vi "ConfigDMM.vi"(8 "error in (no error)":errorcluster, 11 "Input parameters":T1={"Measurement type"=enum."Test", "Sensor type"=enum."HPK_8in_256", "Identifier"="test.txt", "Open after execution?"=FALSE, "Plot after execution?"=FALSE, "Display channel"=0, "Voltage Delay (s)"=0.5, "Switch Delay (s)"=0.01, "VISA resource name source"="", "VISA resource name DMM"="", "VISA resource name LCR"="", "Compliance  Level (uA)"=10.0, "Voltage Limit (V)"=1000.0, "Data storage location"="", "Scan voltages"="", "Use source as DMM?"=FALSE, "Single channel?"=FALSE, "LCR signal frequenzy (Hz)"=10.0, "DMM device"=enum."Keithley2001", "Sampling number"=1, "Use env. sensors on"=enum."Sensirion sht1x/7x"} {"Voltage Limit (V)" format="%#_13g"; "Voltage Delay (s)" format="%#_13g"; "Switch Delay (s)" format="%#_13g"}) -> (0 "error out":errorcluster)   [LabVIEW 2016]
uses:
  Input_parameters.ctl
  instr.lib/ke2001/KE2001.LLB/Keith 2001 Reset / Preset.vi
  instr.lib/Keithley 2450/Keithley 2450.lvlib
panel:
  out "VISA resource name out":refnum<visa-resource-name>
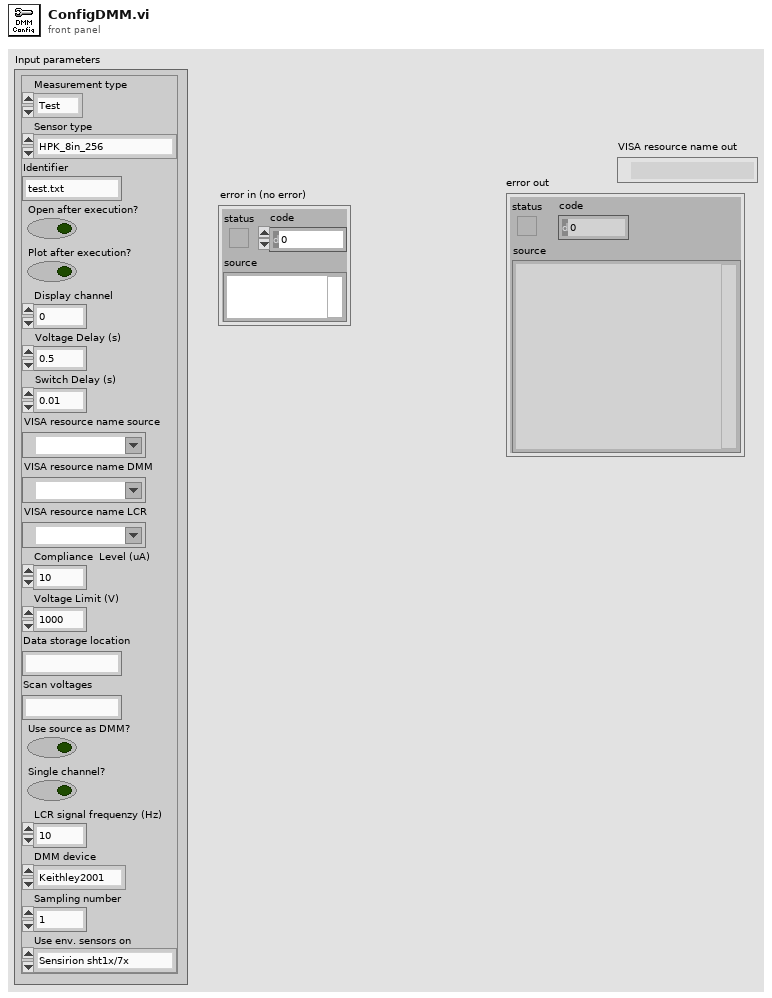
[diagram p1: front panel]
types:
  T1 = typedef "Input_parameters.ctl" = cluster{"Measurement type":enum16{"IV", "CV", "Test"}, "Sensor type":enum16{"HPK_6in_135", "HPK_8in_256", "INF_8in_256", "Diode", "HPK_6in_256", "Test capacitances"}, "Identifier":string, "Open after execution?":bool, "Plot after execution?":bool, "Display channel":i32, "Voltage Delay (s)":dbl, "Switch Delay (s)":dbl, "VISA resource name source":refnum<visa-resource-name>, "VISA resource name DMM":refnum<visa-resource-name>, "VISA resource name LCR":refnum<visa-resource-name>, "Compliance  Level (uA)":dbl, "Voltage Limit (V)":dbl, "Data storage location":string, "Scan voltages":string, "Use source as DMM?":bool, "Single channel?":bool, "LCR signal frequenzy (Hz)":dbl, "DMM device":enum16{"Keithley2001", "Keithley2450", "Keithley2410", "Keithley6487"}, "Sampling number":i32, "Use env. sensors on":enum16{"Sensirion sht1x/7x", "Switch Matrix", "Probecard"}}
  T2 = enum16{"Keithley2001", "Keithley2450", "Keithley2410", "Keithley6487"}
  T3 = enum16{"Auto On", "2e-9", "2e-8", "2e-7", "2e-6", "2e-5", "2e-4", "2e-3", "2e-2"}
  T4 = cluster{"error":bool, "code":i32, "source":string}
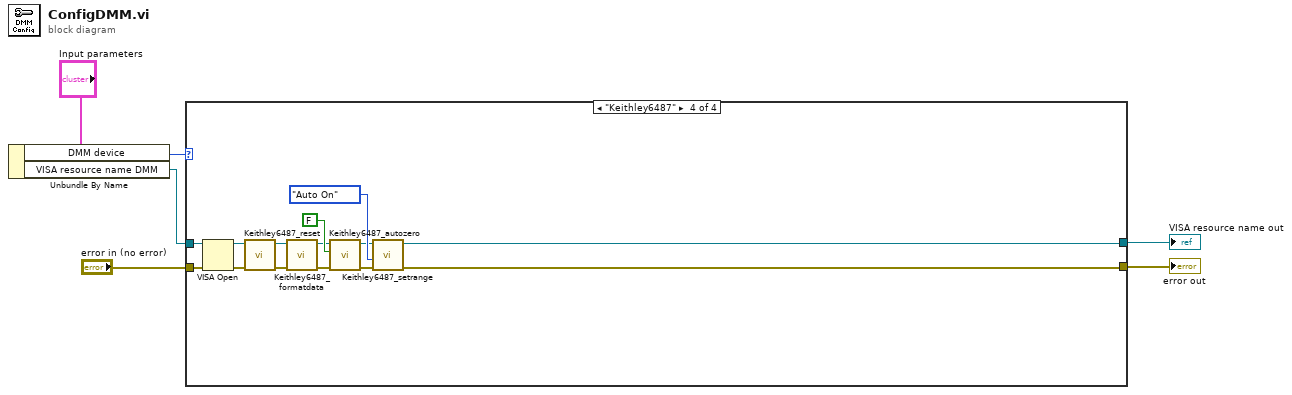
[diagram p0: block diagram]
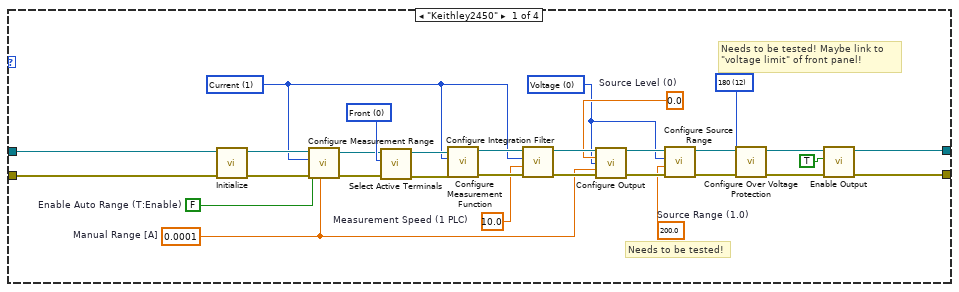
[diagram p2: hidden frame]
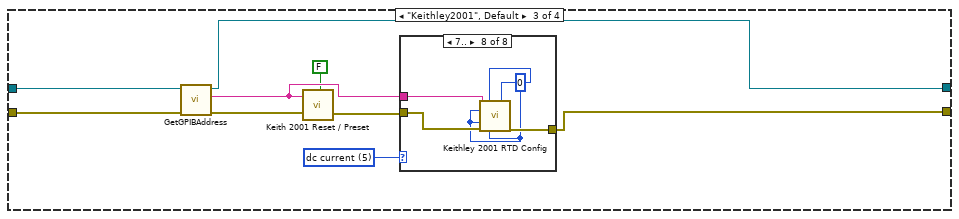
[diagram p4: hidden frame]
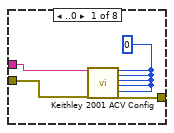
[diagram p5: hidden frame]
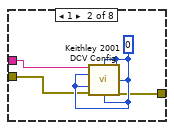
[diagram p6: hidden frame]
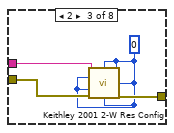
[diagram p7: hidden frame]
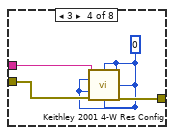
[diagram p8: hidden frame]
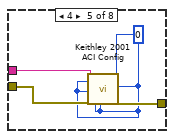
[diagram p9: hidden frame]
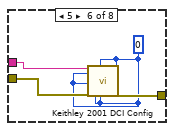
[diagram p10: hidden frame]
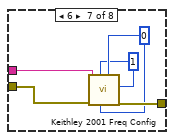
[diagram p11: hidden frame]
diagram:
  n1 = Unbundle By Name("Input parameters") -> ("DMM device"=w3:T2, "VISA resource name DMM"=w2:refnum<visa-resource-name>)
  n2 = case shown="\"Keithley6487\"" w3 {
    tunnel: w2 -> [w36 w38 w45 w83]
    tunnel: "error in (no error)" -> [w35 w37 w44 w84]
    tunnel: [w7 w37 w46 w85] -> w5
    tunnel: [w8 w38 w43 w86] -> w4
    frame "Keithley2450" {
      w12 = u16 12 items=["None", "2", "5", "10", "20", "40", "60", "80", "100", "120", "140", "160", "180"] ("Voltage Limit (0)")
      w15 = 200.0  # Source Range (1.0)
      w20 = 0.0  # Source Level (0)
      w16 = u16 0 items=["Voltage", "Current"] ("Source Mode  (0: Voltage)")
      w23 = 10.0  # Measurement Speed (1 PLC)
      w24 = u16 1 items=["Volts", "Current", "Resistance"] ("Function (0: Volts)")
      w19 = 0.0001  # Manual Range [A]
      w27 = FALSE  # Enable Auto Range (T:Enable)
      w32 = u16 0 items=["Front", "Rear"] ("Active Terminals (0: Front)")
      # "Needs to be tested! Maybe link to \n\"voltage limit\" of front panel!"
      # "Needs to be tested!"
      n3 = call "Initialize.vi"("error in (no error)"=w35, "VISA resource name"=w36) -> ("error out"=w33:errorcluster, "VISA resource name out"=w34:refnum<visa-resource-name>)  [unwired: 8 in]
      n4 = call "Configure Measurement Range.vi"("Manual Range (1.0)"=w19, "error in (no error)"=w33, "Enable Auto Range (T:Enable)"=w27, "Function (0: Volts)"=w24, "VISA resource name"=w34) -> ("error out"=w31:errorcluster, "VISA resource name out"=w28:refnum<visa-resource-name>)  [unwired: 5 in]
      n5 = call "Select Active Terminals.vi"("error in (no error)"=w31, "Active Terminals (0: Front)"=w32, "VISA resource name"=w28) -> ("error out"=w30:errorcluster, "VISA resource name out"=w29:refnum<visa-resource-name>)  [unwired: 7 in]
      n6 = call "Configure Measurement Function.vi"("error in (no error)"=w30, "Function (0: Volts)"=w24, "VISA resource name"=w29) -> ("error out"=w25:errorcluster, "VISA resource name out"=w26:refnum<visa-resource-name>)  [unwired: 7 in]
      n7 = call "Configure Integration Filter.vi"("error in (no error)"=w25, "Measurement Speed (1 PLC)"=w23, "Function (0: Volts)"=w24, "VISA resource name"=w26) -> ("error out"=w21:errorcluster, "VISA resource name out"=w22:refnum<visa-resource-name>)  [unwired: 6 in]
      n8 = call "Configure Output.vi"("VISA resource name"=w22, "Source Level (0)"=w20, "Source Mode  (0: Voltage)"=w16, "Source Limit Level (0.1)"=w19, "error in (no error)"=w21) -> ("VISA resource name out"=w17:refnum<visa-resource-name>, "error out"=w18:errorcluster)  [unwired: 9 in]
      n9 = call "Configure Source Range.vi"("error in (no error)"=w18, "Source Range (1.0)"=w15, "Function (0: Volts)"=w16, "VISA resource name"=w17) -> ("error out"=w14:errorcluster, "VISA resource name out"=w13:refnum<visa-resource-name>)  [unwired: 6 in]
      n10 = call "Configure Over Voltage Protection.vi"("error in (no error)"=w14, "Voltage Limit (0)"=w12, "VISA resource name"=w13) -> ("error out"=w10:errorcluster, "VISA resource name out"=w9:refnum<visa-resource-name>)  [unwired: 7 in]
      n11 = call "Enable Output.vi"("error in (no error)"=w10, "Enable Output (T: Enable)"=TRUE, "VISA resource name"=w9) -> ("error out"=w7:errorcluster, "VISA resource name out"=w8:refnum<visa-resource-name>)  [unwired: 7 in]
    }
    frame "Keithley2410" {
    }
    frame "Keithley2001", Default {
      w47 = u16 5 items=["ac voltage", "dc voltage", "2-wire resistance", "4-wire resistance", "ac current", "dc current", "frequency", "temperature"] ("function (Vdc:1)")
      n12 = call "GetGPIBAddress.vi"("error in (no error)"=w44, "VISA resource name"=w45) -> ("error out"=w42:errorcluster, "GPIB address"=w41:string, "VISA resource name out"=w43:refnum<visa-resource-name>)  [unwired: 7 in]
      n13 = call "Keith 2001 Reset / Preset.vi"("reset/preset"=FALSE, "error in"=w42, "GPIB address"=w41) -> ("error out"=w40:T4)
      n14 = case shown="7.." w47 {
        tunnel: w40 -> [w50 w54 w58 w62 w66 w70 w75 w79]
        tunnel: w41 -> [w48 w53 w57 w61 w65 w68 w74 w78]
        tunnel: [w49 w52 w59 w63 w67 w71 w76 w80] -> w46
        frame ..0 {
          w51 = u16 0
          n15 = call "Keithley 2001 ACV Config.vi"("GPIB address"=w48, "integration time (0:auto)"=w51, "integ. value"=w51, "range (auto:0)"=w51, "error in"=w50, "resolution (4.5 digits:3)"=w51, "reference (off:0)"=w51, "digital filter (off:0)"=w51, "advanced filter (off:0)"=w51, "detector (rms:0)"=w51) -> ("error out"=w49:T4)  [unwired: 9 in]
        }
        frame 1 {
          w55 = u16 0
          n16 = call "Keithley 2001 DCV Config.vi"("GPIB address"=w53, "range (auto:0)"=w55, "digital filter (off:0)"=w55, "integration time (0:auto)"=w55, "advanced filter (off:0)"=w55, "resolution (4.5 digits:3)"=w55, "error in"=w54, "reference value (volts)"=w55) -> ("error out"=w52:T4)  [unwired: 7 in]
        }
        frame 2 {
          w56 = u16 0
          n17 = call "Keithley 2001 2-W Res Config.vi"("GPIB address"=w57, "range (auto:0)"=w56, "digital filter (off:0)"=w56, "integration time (0:auto)"=w56, "advanced filter (off:0)"=w56, "resolution (4.5 digits:3)"=w56, "error in"=w58, "reference value (ohms)"=w56) -> ("error out"=w59:T4)  [unwired: 7 in]
        }
        frame 3 {
          w60 = u16 0
          n18 = call "Keithley 2001 4-W Res Config.vi"("GPIB address"=w61, "range (auto:0)"=w60, "digital filter (off:0)"=w60, "integration time (0:auto)"=w60, "advanced filter (off:0)"=w60, "resolution (4.5 digits:3)"=w60, "error in"=w62, "reference value (ohms)"=w60) -> ("error out"=w63:T4)  [unwired: 7 in]
        }
        frame 4 {
          w64 = u16 0
          n19 = call "Keithley 2001 ACI Config.vi"("GPIB address"=w65, "integration time (0:auto)"=w64, "range (auto:0)"=w64, "error in"=w66, "resolution (4.5 digits:3)"=w64, "digital filter (off:0)"=w64, "advanced filter (off:0)"=w64, "detector (rms:0)"=w64) -> ("error out"=w67:T4)  [unwired: 11 in]
        }
        frame 5 {
          w69 = u16 0
          n20 = call "Keithley 2001 DCI Config.vi"("GPIB address"=w68, "integration time (0:auto)"=w69, "range (auto:0)"=w69, "error in"=w70, "resolution (4.5 digits:3)"=w69, "reference (off:0)"=w69, "digital filter (off:0)"=w69, "advanced filter (off:0)"=w69) -> ("error out"=w71:T4)  [unwired: 11 in]
        }
        frame 6 {
          w72 = u16 1
          w73 = u16 0
          n21 = call "Keithley 2001 Freq Config.vi"("threshold voltage range (10V:1)"=w72, "threshold current range (1mA:0)"=w73, "reference (off:0)"=w73, "resolution (5 digits:1)"=w72, "error in"=w75, "GPIB address"=w74) -> ("error out"=w76:T4)  [unwired: 5 in]
        }
        frame 7.. {
          w77 = u16 0
          n22 = call "Keithley 2001 RTD Config.vi"("GPIB address"=w78, "reference (off:0)"=w77, "transducer (2-W RTD-PT385:0)"=w77, "integration time (0:auto)"=w77, "resolution (5.5 digits:4)"=w77, "error in"=w79, "digital filter (off:0)"=w77) -> ("error out"=w80:T4)  [unwired: 8 in]
        }
      }
    }
    frame "Keithley6487" {
      n23 = VISA Open(error in (no error)=w84, VISA resource name=w83) -> (VISA resource name=w82:refnum<visa-resource-name>, error out=w81:errorcluster)  [unwired: 3 in]
      n24 = call "Keithley6487_reset.vi"("error in (no error)"=w81, "VISA resource name"=w82) -> ("error out"=w92:errorcluster, "VISA resource name out"=w89:refnum<visa-resource-name>)  [unwired: 8 in]
      n25 = call "Keithley6487_formatdata.vi"("error in (no error)"=w92, "VISA resource name"=w89) -> ("error out"=w91:errorcluster, "VISA resource name out"=w88:refnum<visa-resource-name>)  [unwired: 8 in]
      n26 = call "Keithley6487_autozero.vi"("error in (no error)"=w91, "Autozero"=FALSE, "VISA resource name"=w88) -> ("error out"=w90:errorcluster, "VISA resource name out"=w87:refnum<visa-resource-name>)  [unwired: 7 in]
      n27 = call "Keithley6487_setrange.vi"("error in (no error)"=w90, "Enum"=T3."Auto On", "VISA resource name"=w87) -> ("error out"=w85:errorcluster, "VISA resource name out"=w86:refnum<visa-resource-name>)  [unwired: 7 in]
    }
  }
  "VISA resource name out" <- w4
  "error out" <- w5
